vi "Unicode List Folder Example.vi"() -> ()   [LabVIEW 2020]
uses:
  Types/UTF-8 String/UTF-8 String.lvclass/UTF-8 String.ctl
  Types/UTF-8 Path/UTF-8 Path.lvclass/UTF-8 Path.ctl
  356e65d8-4da9-4114-9294-e55a313f9948.vi
  39fc5e22-d9af-4d01-836e-3ce06c2f0119.vi
  9656b7da-fab8-46cb-9ac0-8f81757845da.vi
  0798be5a-71d1-4c5d-88ab-63fcb16b67de.vi
  333a896f-bbc2-4275-b957-7d35ff018cee.vi
  d770f125-4b2e-45a9-bf4a-bdfa33aeb32b.vi
  be28db5e-b7b6-4e5e-976e-8f4788af5f3e.vi
  d890a278-da3a-47ea-bd3f-d0f581a9f8a0.vi
  e6b5bfce-c779-4612-a132-177d94a25bbe.vi
  cbe0ae27-dce3-42f5-8311-771008e4fc32.vi
  faa403f0-121f-4031-81ad-bed2ef2c299f.vi
  9acd3354-284c-4284-bd8f-25762292fedc.vi
  356e65d8-4da9-4114-9294-e55a313f9948.vi/394fe735-5a0a-4c6e-b10c-ef5f4bad8cdd.vi
  356e65d8-4da9-4114-9294-e55a313f9948.vi/c6ff4536-5c5f-4898-b0f4-ba79e0235d06.vi
  Private/Conversion/String as Encoded String.vi
  Private/Conversion/Polymorphic VIs/String as Encoded String (UTF-8 String).vi
  Types/UTF-8 String/Write Encoded UTF-8 String.vi
  39fc5e22-d9af-4d01-836e-3ce06c2f0119.vi/9afeabe8-8abe-4536-bea1-05e5a3549c28.vi
  Private/Conversion/Text as Encoded String.vi
  Private/Conversion/Polymorphic VIs/Text as Encoded String (UTF-8 String).vi
  Private/Library/gu_open_file_dialog.vi
  Private/Library/gu_select_folder_dialog.vi
  9656b7da-fab8-46cb-9ac0-8f81757845da.vi/5206cb6b-04fb-41f5-a37e-29c14f142303.vi
  0798be5a-71d1-4c5d-88ab-63fcb16b67de.vi/394fe735-5a0a-4c6e-b10c-ef5f4bad8cdd.vi
  0798be5a-71d1-4c5d-88ab-63fcb16b67de.vi/c6ff4536-5c5f-4898-b0f4-ba79e0235d06.vi
  Private/Conversion/Text as String.vi
  Private/Conversion/Polymorphic VIs/Text as String (UTF-8 String).vi
  Private/Conversion/Text as Encoded Path.vi
  Private/Conversion/Polymorphic VIs/Text as Encoded Path (UTF-8 String).vi
  Types/UTF-8 Path/Write Encoded UTF-8 Path.vi
  Private/Conversion/Path as UTF-8 Path.vi
  Private/Conversion/Polymorphic VIs/Path as UTF-8 Path (UTF-8 Path).vi
  be28db5e-b7b6-4e5e-976e-8f4788af5f3e.vi/5269e09c-4216-478e-8686-9fb7d38e224a.vi
  be28db5e-b7b6-4e5e-976e-8f4788af5f3e.vi/d1f4a45d-6f02-44dd-a40b-2b28d80e6519.vi
  Private/Library/gu_list_folder.vi
  be28db5e-b7b6-4e5e-976e-8f4788af5f3e.vi/8eb4f0ed-0012-4550-978e-be3f7301df70.vi
  be28db5e-b7b6-4e5e-976e-8f4788af5f3e.vi/f7e6584c-01ed-423f-9bcd-660954191d0d.vi
  d890a278-da3a-47ea-bd3f-d0f581a9f8a0.vi/00b95b8e-259c-4cd2-84a0-259870334f57.vi
  d890a278-da3a-47ea-bd3f-d0f581a9f8a0.vi/6e4bb66e-265d-408c-9dfe-e7c3a7878e52.vi
  d890a278-da3a-47ea-bd3f-d0f581a9f8a0.vi/08f180d4-fb41-400e-a869-abb2918b55f1.vi
  d890a278-da3a-47ea-bd3f-d0f581a9f8a0.vi/5ea8612d-ac84-4b15-a8e8-3f95405e799f.vi
  d890a278-da3a-47ea-bd3f-d0f581a9f8a0.vi/f443e8ba-b003-43b4-b0bc-fd2b779e8587.vi
  d890a278-da3a-47ea-bd3f-d0f581a9f8a0.vi/c6b89822-a9c0-4fa9-a4a0-f7d505b8bbe9.vi
  d890a278-da3a-47ea-bd3f-d0f581a9f8a0.vi/54676e99-5528-43ca-932e-9ead8464c752.vi
  d890a278-da3a-47ea-bd3f-d0f581a9f8a0.vi/9bf89ca9-aafa-4aa0-9117-a6707f6e0e94.vi
  d890a278-da3a-47ea-bd3f-d0f581a9f8a0.vi/e7542c1a-d99f-41ff-9d9a-3ecd282cacf4.vi
  d890a278-da3a-47ea-bd3f-d0f581a9f8a0.vi/d8f6ae1f-7202-4db9-b87a-1f416505b7ed.vi
  Private/Conversion/Polymorphic VIs/Text as Encoded String (UTF-8 Path).vi
  faa403f0-121f-4031-81ad-bed2ef2c299f.vi/5206cb6b-04fb-41f5-a37e-29c14f142303.vi
  9acd3354-284c-4284-bd8f-25762292fedc.vi/5206cb6b-04fb-41f5-a37e-29c14f142303.vi
  Private/Conversion/String as UTF-8 String.vi
  Private/Conversion/Polymorphic VIs/String as UTF-8 String (LabVIEW String).vi
  Types/UTF-8 String/Read Encoded UTF-8 String.vi
  Private/Memory/Copy String.vi
  Private/Library/Result To Error.vi
  be28db5e-b7b6-4e5e-976e-8f4788af5f3e.vi/5269e09c-4216-478e-8686-9fb7d38e224a.vi/c24c063b-f849-48a1-b323-238a063d7118.vi
  be28db5e-b7b6-4e5e-976e-8f4788af5f3e.vi/5269e09c-4216-478e-8686-9fb7d38e224a.vi/a2fd6c11-d594-45c9-8624-1f0a1df69df3.vi
  be28db5e-b7b6-4e5e-976e-8f4788af5f3e.vi/5269e09c-4216-478e-8686-9fb7d38e224a.vi/1fd3173e-d32e-42cb-8f0d-819132eb8e27.vi
  be28db5e-b7b6-4e5e-976e-8f4788af5f3e.vi/5269e09c-4216-478e-8686-9fb7d38e224a.vi/bb7c39fc-ad8e-447d-bc50-468674bfb562.vi
  be28db5e-b7b6-4e5e-976e-8f4788af5f3e.vi/8eb4f0ed-0012-4550-978e-be3f7301df70.vi/3a31b270-3bb6-4c58-a256-c5fcc2c98f09.vi
  be28db5e-b7b6-4e5e-976e-8f4788af5f3e.vi/8eb4f0ed-0012-4550-978e-be3f7301df70.vi/0ec5df2d-ef9b-4f84-a6a8-ffcedd45c4dc.vi
  Private/Conversion/Polymorphic VIs/Text as String (UTF-8 Path).vi
  Private/Conversion/Path as Encoded Path.vi
  Private/Conversion/Polymorphic VIs/Path as Encoded Path (UTF-8 Path).vi
  Private/Library/gu_to_lower_case.vi
  d890a278-da3a-47ea-bd3f-d0f581a9f8a0.vi/08f180d4-fb41-400e-a869-abb2918b55f1.vi/5269e09c-4216-478e-8686-9fb7d38e224a.vi
  d890a278-da3a-47ea-bd3f-d0f581a9f8a0.vi/08f180d4-fb41-400e-a869-abb2918b55f1.vi/d1f4a45d-6f02-44dd-a40b-2b28d80e6519.vi
  d890a278-da3a-47ea-bd3f-d0f581a9f8a0.vi/08f180d4-fb41-400e-a869-abb2918b55f1.vi/8eb4f0ed-0012-4550-978e-be3f7301df70.vi
  d890a278-da3a-47ea-bd3f-d0f581a9f8a0.vi/08f180d4-fb41-400e-a869-abb2918b55f1.vi/f7e6584c-01ed-423f-9bcd-660954191d0d.vi
  d890a278-da3a-47ea-bd3f-d0f581a9f8a0.vi/5ea8612d-ac84-4b15-a8e8-3f95405e799f.vi/5269e09c-4216-478e-8686-9fb7d38e224a.vi
  d890a278-da3a-47ea-bd3f-d0f581a9f8a0.vi/5ea8612d-ac84-4b15-a8e8-3f95405e799f.vi/d1f4a45d-6f02-44dd-a40b-2b28d80e6519.vi
  d890a278-da3a-47ea-bd3f-d0f581a9f8a0.vi/5ea8612d-ac84-4b15-a8e8-3f95405e799f.vi/8eb4f0ed-0012-4550-978e-be3f7301df70.vi
  d890a278-da3a-47ea-bd3f-d0f581a9f8a0.vi/5ea8612d-ac84-4b15-a8e8-3f95405e799f.vi/f7e6584c-01ed-423f-9bcd-660954191d0d.vi
  d890a278-da3a-47ea-bd3f-d0f581a9f8a0.vi/f443e8ba-b003-43b4-b0bc-fd2b779e8587.vi/bdbb2850-443b-457b-baea-a8ca465ac309.vi
  d890a278-da3a-47ea-bd3f-d0f581a9f8a0.vi/f443e8ba-b003-43b4-b0bc-fd2b779e8587.vi/12c50203-b387-4b7f-a219-1cc37bee024e.vi
  d890a278-da3a-47ea-bd3f-d0f581a9f8a0.vi/f443e8ba-b003-43b4-b0bc-fd2b779e8587.vi/79db7a21-11bb-4b22-98c5-d1966ec86c45.vi
  d890a278-da3a-47ea-bd3f-d0f581a9f8a0.vi/f443e8ba-b003-43b4-b0bc-fd2b779e8587.vi/90888b97-91dc-4a8b-9ef5-bc117a67dfd4.vi
  d890a278-da3a-47ea-bd3f-d0f581a9f8a0.vi/f443e8ba-b003-43b4-b0bc-fd2b779e8587.vi/1e320fb2-7d21-4fd0-8d77-02d925575486.vi
  d890a278-da3a-47ea-bd3f-d0f581a9f8a0.vi/f443e8ba-b003-43b4-b0bc-fd2b779e8587.vi/3a50a1cc-fee8-47d0-b63a-e1c29b38961d.vi
  d890a278-da3a-47ea-bd3f-d0f581a9f8a0.vi/54676e99-5528-43ca-932e-9ead8464c752.vi/4d3f9d4a-5006-44fd-9ac3-fe6a2ce0b86b.vi
  d890a278-da3a-47ea-bd3f-d0f581a9f8a0.vi/54676e99-5528-43ca-932e-9ead8464c752.vi/29e5914f-c0b0-4539-b998-9919647c2bfd.vi
  d890a278-da3a-47ea-bd3f-d0f581a9f8a0.vi/9bf89ca9-aafa-4aa0-9117-a6707f6e0e94.vi/4d3f9d4a-5006-44fd-9ac3-fe6a2ce0b86b.vi
  d890a278-da3a-47ea-bd3f-d0f581a9f8a0.vi/9bf89ca9-aafa-4aa0-9117-a6707f6e0e94.vi/29e5914f-c0b0-4539-b998-9919647c2bfd.vi
  Types/UTF-8 Path/Read Encoded UTF-8 Path.vi
  Types/UTF-8 String/New UTF-8 String.vi
  Private/Memory/Copy String.vi/4d47babd-4a2d-4eb7-b91b-7e707d692665.vi
  Private/Library/gu_free.vi
  Private/Library/gu_string_subset.vi
  Private/Library/gu_search_split_string.vi
  Private/Conversion/Polymorphic VIs/String as Encoded String (LabVIEW String).vi
  Private/Conversion/Polymorphic VIs/Text as Encoded String (LabVIEW String).vi
  d890a278-da3a-47ea-bd3f-d0f581a9f8a0.vi/08f180d4-fb41-400e-a869-abb2918b55f1.vi/5269e09c-4216-478e-8686-9fb7d38e224a.vi/c24c063b-f849-48a1-b323-238a063d7118.vi
  d890a278-da3a-47ea-bd3f-d0f581a9f8a0.vi/08f180d4-fb41-400e-a869-abb2918b55f1.vi/5269e09c-4216-478e-8686-9fb7d38e224a.vi/a2fd6c11-d594-45c9-8624-1f0a1df69df3.vi
  d890a278-da3a-47ea-bd3f-d0f581a9f8a0.vi/08f180d4-fb41-400e-a869-abb2918b55f1.vi/5269e09c-4216-478e-8686-9fb7d38e224a.vi/1fd3173e-d32e-42cb-8f0d-819132eb8e27.vi
  d890a278-da3a-47ea-bd3f-d0f581a9f8a0.vi/08f180d4-fb41-400e-a869-abb2918b55f1.vi/5269e09c-4216-478e-8686-9fb7d38e224a.vi/bb7c39fc-ad8e-447d-bc50-468674bfb562.vi
  d890a278-da3a-47ea-bd3f-d0f581a9f8a0.vi/08f180d4-fb41-400e-a869-abb2918b55f1.vi/8eb4f0ed-0012-4550-978e-be3f7301df70.vi/3a31b270-3bb6-4c58-a256-c5fcc2c98f09.vi
  d890a278-da3a-47ea-bd3f-d0f581a9f8a0.vi/08f180d4-fb41-400e-a869-abb2918b55f1.vi/8eb4f0ed-0012-4550-978e-be3f7301df70.vi/0ec5df2d-ef9b-4f84-a6a8-ffcedd45c4dc.vi
  d890a278-da3a-47ea-bd3f-d0f581a9f8a0.vi/5ea8612d-ac84-4b15-a8e8-3f95405e799f.vi/5269e09c-4216-478e-8686-9fb7d38e224a.vi/c24c063b-f849-48a1-b323-238a063d7118.vi
  d890a278-da3a-47ea-bd3f-d0f581a9f8a0.vi/5ea8612d-ac84-4b15-a8e8-3f95405e799f.vi/5269e09c-4216-478e-8686-9fb7d38e224a.vi/a2fd6c11-d594-45c9-8624-1f0a1df69df3.vi
  d890a278-da3a-47ea-bd3f-d0f581a9f8a0.vi/5ea8612d-ac84-4b15-a8e8-3f95405e799f.vi/5269e09c-4216-478e-8686-9fb7d38e224a.vi/1fd3173e-d32e-42cb-8f0d-819132eb8e27.vi
  d890a278-da3a-47ea-bd3f-d0f581a9f8a0.vi/5ea8612d-ac84-4b15-a8e8-3f95405e799f.vi/5269e09c-4216-478e-8686-9fb7d38e224a.vi/bb7c39fc-ad8e-447d-bc50-468674bfb562.vi
  d890a278-da3a-47ea-bd3f-d0f581a9f8a0.vi/5ea8612d-ac84-4b15-a8e8-3f95405e799f.vi/8eb4f0ed-0012-4550-978e-be3f7301df70.vi/3a31b270-3bb6-4c58-a256-c5fcc2c98f09.vi
  d890a278-da3a-47ea-bd3f-d0f581a9f8a0.vi/5ea8612d-ac84-4b15-a8e8-3f95405e799f.vi/8eb4f0ed-0012-4550-978e-be3f7301df70.vi/0ec5df2d-ef9b-4f84-a6a8-ffcedd45c4dc.vi
  d890a278-da3a-47ea-bd3f-d0f581a9f8a0.vi/f443e8ba-b003-43b4-b0bc-fd2b779e8587.vi/90888b97-91dc-4a8b-9ef5-bc117a67dfd4.vi/5269e09c-4216-478e-8686-9fb7d38e224a.vi
  d890a278-da3a-47ea-bd3f-d0f581a9f8a0.vi/f443e8ba-b003-43b4-b0bc-fd2b779e8587.vi/90888b97-91dc-4a8b-9ef5-bc117a67dfd4.vi/d1f4a45d-6f02-44dd-a40b-2b28d80e6519.vi
  d890a278-da3a-47ea-bd3f-d0f581a9f8a0.vi/f443e8ba-b003-43b4-b0bc-fd2b779e8587.vi/90888b97-91dc-4a8b-9ef5-bc117a67dfd4.vi/8eb4f0ed-0012-4550-978e-be3f7301df70.vi
  d890a278-da3a-47ea-bd3f-d0f581a9f8a0.vi/f443e8ba-b003-43b4-b0bc-fd2b779e8587.vi/90888b97-91dc-4a8b-9ef5-bc117a67dfd4.vi/f7e6584c-01ed-423f-9bcd-660954191d0d.vi
  d890a278-da3a-47ea-bd3f-d0f581a9f8a0.vi/f443e8ba-b003-43b4-b0bc-fd2b779e8587.vi/1e320fb2-7d21-4fd0-8d77-02d925575486.vi/5269e09c-4216-478e-8686-9fb7d38e224a.vi
  d890a278-da3a-47ea-bd3f-d0f581a9f8a0.vi/f443e8ba-b003-43b4-b0bc-fd2b779e8587.vi/1e320fb2-7d21-4fd0-8d77-02d925575486.vi/d1f4a45d-6f02-44dd-a40b-2b28d80e6519.vi
  d890a278-da3a-47ea-bd3f-d0f581a9f8a0.vi/f443e8ba-b003-43b4-b0bc-fd2b779e8587.vi/1e320fb2-7d21-4fd0-8d77-02d925575486.vi/8eb4f0ed-0012-4550-978e-be3f7301df70.vi
  d890a278-da3a-47ea-bd3f-d0f581a9f8a0.vi/f443e8ba-b003-43b4-b0bc-fd2b779e8587.vi/1e320fb2-7d21-4fd0-8d77-02d925575486.vi/f7e6584c-01ed-423f-9bcd-660954191d0d.vi
  d890a278-da3a-47ea-bd3f-d0f581a9f8a0.vi/f443e8ba-b003-43b4-b0bc-fd2b779e8587.vi/3a50a1cc-fee8-47d0-b63a-e1c29b38961d.vi/5269e09c-4216-478e-8686-9fb7d38e224a.vi
  d890a278-da3a-47ea-bd3f-d0f581a9f8a0.vi/f443e8ba-b003-43b4-b0bc-fd2b779e8587.vi/3a50a1cc-fee8-47d0-b63a-e1c29b38961d.vi/d1f4a45d-6f02-44dd-a40b-2b28d80e6519.vi
  d890a278-da3a-47ea-bd3f-d0f581a9f8a0.vi/f443e8ba-b003-43b4-b0bc-fd2b779e8587.vi/3a50a1cc-fee8-47d0-b63a-e1c29b38961d.vi/8eb4f0ed-0012-4550-978e-be3f7301df70.vi
  d890a278-da3a-47ea-bd3f-d0f581a9f8a0.vi/f443e8ba-b003-43b4-b0bc-fd2b779e8587.vi/3a50a1cc-fee8-47d0-b63a-e1c29b38961d.vi/f7e6584c-01ed-423f-9bcd-660954191d0d.vi
  Private/Conversion/Text to UTF-8.vi
  Private/Conversion/Polymorphic VIs/Text to UTF-8 (LabVIEW String).vi
  d890a278-da3a-47ea-bd3f-d0f581a9f8a0.vi/f443e8ba-b003-43b4-b0bc-fd2b779e8587.vi/90888b97-91dc-4a8b-9ef5-bc117a67dfd4.vi/5269e09c-4216-478e-8686-9fb7d38e224a.vi/c24c063b-f849-48a1-b323-238a063d7118.vi
  d890a278-da3a-47ea-bd3f-d0f581a9f8a0.vi/f443e8ba-b003-43b4-b0bc-fd2b779e8587.vi/90888b97-91dc-4a8b-9ef5-bc117a67dfd4.vi/5269e09c-4216-478e-8686-9fb7d38e224a.vi/a2fd6c11-d594-45c9-8624-1f0a1df69df3.vi
  d890a278-da3a-47ea-bd3f-d0f581a9f8a0.vi/f443e8ba-b003-43b4-b0bc-fd2b779e8587.vi/90888b97-91dc-4a8b-9ef5-bc117a67dfd4.vi/5269e09c-4216-478e-8686-9fb7d38e224a.vi/1fd3173e-d32e-42cb-8f0d-819132eb8e27.vi
  d890a278-da3a-47ea-bd3f-d0f581a9f8a0.vi/f443e8ba-b003-43b4-b0bc-fd2b779e8587.vi/90888b97-91dc-4a8b-9ef5-bc117a67dfd4.vi/5269e09c-4216-478e-8686-9fb7d38e224a.vi/bb7c39fc-ad8e-447d-bc50-468674bfb562.vi
  d890a278-da3a-47ea-bd3f-d0f581a9f8a0.vi/f443e8ba-b003-43b4-b0bc-fd2b779e8587.vi/90888b97-91dc-4a8b-9ef5-bc117a67dfd4.vi/8eb4f0ed-0012-4550-978e-be3f7301df70.vi/3a31b270-3bb6-4c58-a256-c5fcc2c98f09.vi
  d890a278-da3a-47ea-bd3f-d0f581a9f8a0.vi/f443e8ba-b003-43b4-b0bc-fd2b779e8587.vi/90888b97-91dc-4a8b-9ef5-bc117a67dfd4.vi/8eb4f0ed-0012-4550-978e-be3f7301df70.vi/0ec5df2d-ef9b-4f84-a6a8-ffcedd45c4dc.vi
  d890a278-da3a-47ea-bd3f-d0f581a9f8a0.vi/f443e8ba-b003-43b4-b0bc-fd2b779e8587.vi/1e320fb2-7d21-4fd0-8d77-02d925575486.vi/5269e09c-4216-478e-8686-9fb7d38e224a.vi/c24c063b-f849-48a1-b323-238a063d7118.vi
  d890a278-da3a-47ea-bd3f-d0f581a9f8a0.vi/f443e8ba-b003-43b4-b0bc-fd2b779e8587.vi/1e320fb2-7d21-4fd0-8d77-02d925575486.vi/5269e09c-4216-478e-8686-9fb7d38e224a.vi/a2fd6c11-d594-45c9-8624-1f0a1df69df3.vi
  d890a278-da3a-47ea-bd3f-d0f581a9f8a0.vi/f443e8ba-b003-43b4-b0bc-fd2b779e8587.vi/1e320fb2-7d21-4fd0-8d77-02d925575486.vi/5269e09c-4216-478e-8686-9fb7d38e224a.vi/1fd3173e-d32e-42cb-8f0d-819132eb8e27.vi
  d890a278-da3a-47ea-bd3f-d0f581a9f8a0.vi/f443e8ba-b003-43b4-b0bc-fd2b779e8587.vi/1e320fb2-7d21-4fd0-8d77-02d925575486.vi/5269e09c-4216-478e-8686-9fb7d38e224a.vi/bb7c39fc-ad8e-447d-bc50-468674bfb562.vi
  d890a278-da3a-47ea-bd3f-d0f581a9f8a0.vi/f443e8ba-b003-43b4-b0bc-fd2b779e8587.vi/1e320fb2-7d21-4fd0-8d77-02d925575486.vi/8eb4f0ed-0012-4550-978e-be3f7301df70.vi/3a31b270-3bb6-4c58-a256-c5fcc2c98f09.vi
  d890a278-da3a-47ea-bd3f-d0f581a9f8a0.vi/f443e8ba-b003-43b4-b0bc-fd2b779e8587.vi/1e320fb2-7d21-4fd0-8d77-02d925575486.vi/8eb4f0ed-0012-4550-978e-be3f7301df70.vi/0ec5df2d-ef9b-4f84-a6a8-ffcedd45c4dc.vi
  d890a278-da3a-47ea-bd3f-d0f581a9f8a0.vi/f443e8ba-b003-43b4-b0bc-fd2b779e8587.vi/3a50a1cc-fee8-47d0-b63a-e1c29b38961d.vi/5269e09c-4216-478e-8686-9fb7d38e224a.vi/c24c063b-f849-48a1-b323-238a063d7118.vi
  d890a278-da3a-47ea-bd3f-d0f581a9f8a0.vi/f443e8ba-b003-43b4-b0bc-fd2b779e8587.vi/3a50a1cc-fee8-47d0-b63a-e1c29b38961d.vi/5269e09c-4216-478e-8686-9fb7d38e224a.vi/a2fd6c11-d594-45c9-8624-1f0a1df69df3.vi
  d890a278-da3a-47ea-bd3f-d0f581a9f8a0.vi/f443e8ba-b003-43b4-b0bc-fd2b779e8587.vi/3a50a1cc-fee8-47d0-b63a-e1c29b38961d.vi/5269e09c-4216-478e-8686-9fb7d38e224a.vi/1fd3173e-d32e-42cb-8f0d-819132eb8e27.vi
  d890a278-da3a-47ea-bd3f-d0f581a9f8a0.vi/f443e8ba-b003-43b4-b0bc-fd2b779e8587.vi/3a50a1cc-fee8-47d0-b63a-e1c29b38961d.vi/5269e09c-4216-478e-8686-9fb7d38e224a.vi/bb7c39fc-ad8e-447d-bc50-468674bfb562.vi
  d890a278-da3a-47ea-bd3f-d0f581a9f8a0.vi/f443e8ba-b003-43b4-b0bc-fd2b779e8587.vi/3a50a1cc-fee8-47d0-b63a-e1c29b38961d.vi/8eb4f0ed-0012-4550-978e-be3f7301df70.vi/3a31b270-3bb6-4c58-a256-c5fcc2c98f09.vi
  d890a278-da3a-47ea-bd3f-d0f581a9f8a0.vi/f443e8ba-b003-43b4-b0bc-fd2b779e8587.vi/3a50a1cc-fee8-47d0-b63a-e1c29b38961d.vi/8eb4f0ed-0012-4550-978e-be3f7301df70.vi/0ec5df2d-ef9b-4f84-a6a8-ffcedd45c4dc.vi
  Private/User Interface/Read String.vi
  Unicode/Detect String Encoding.vi
  Private/Conversion/Encoded UTF-16LE String to Encoded UTF-8 String.vi
  <vilib>/Utility/error.llb/Error Cluster From Error Code.vi
  Private/Conversion/Encoded UTF-8 String to Encoded UTF-16LE String.vi
  Private/User Interface/Write String.vi
  Private/Memory/Copy String Array.vi
  File IO/Path to Short Name.vi
  Private/Library/gu_strlen.vi
  Private/User Interface/Write String Array (1D).vi
  Types/UTF-8 String/UTF-8 String.lvclass
  Types/UTF-8 Path/UTF-8 Path.lvclass
panel:
  in  "Refresh Button":bool
  in  "Recursive List":bool
  out "Files":string[](array[string])
  out "Folders":string[](array[string])
  in  "Browse Button":bool
  out "Path":string
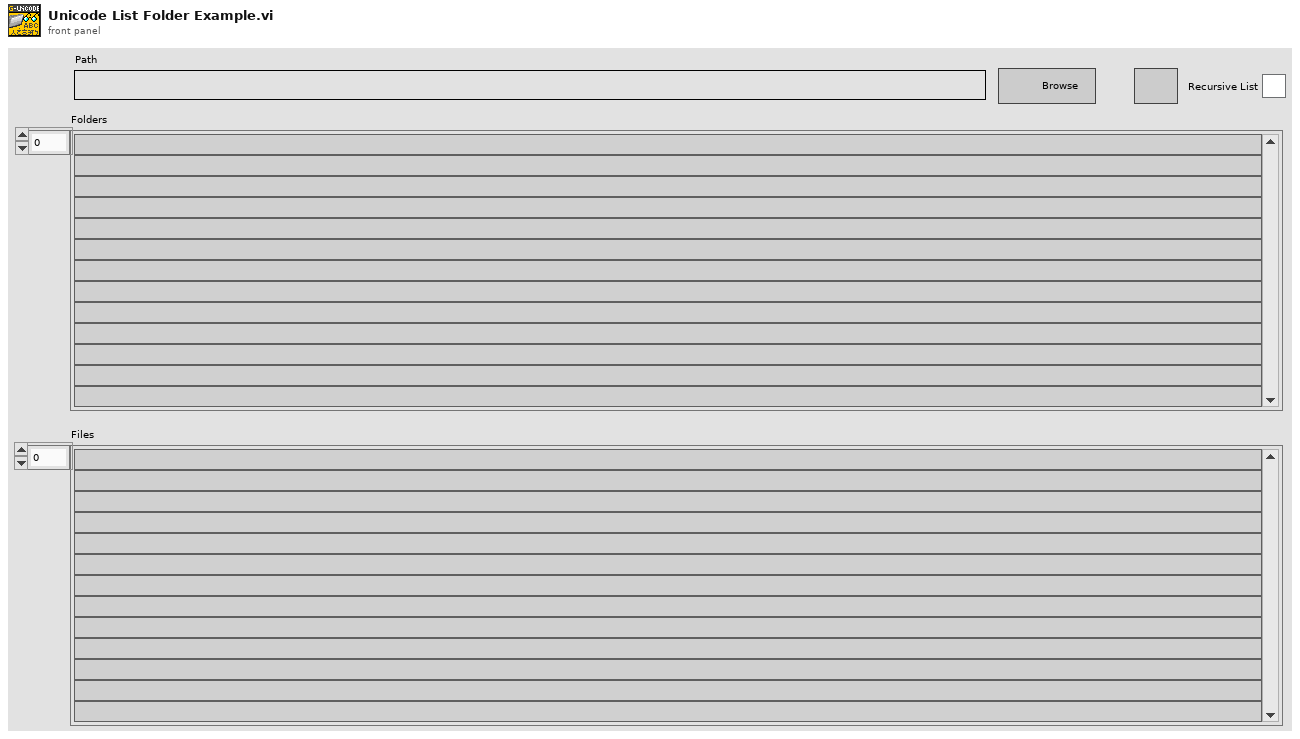
[diagram p1: front panel]
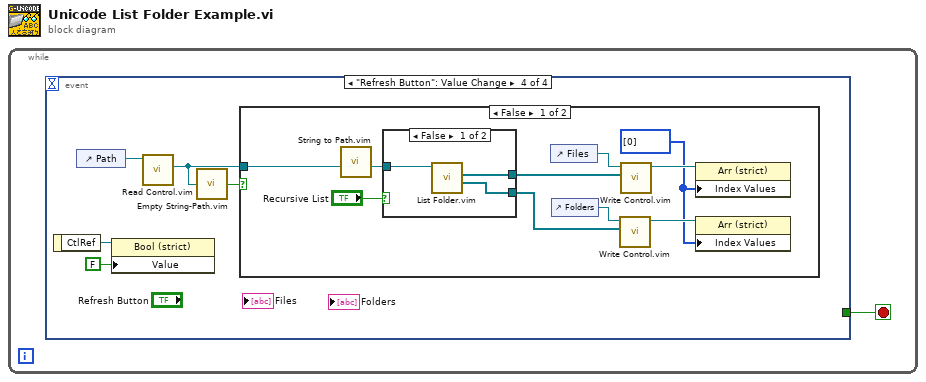
[diagram p0: block diagram]
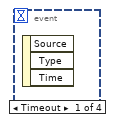
[diagram p2: hidden frame]
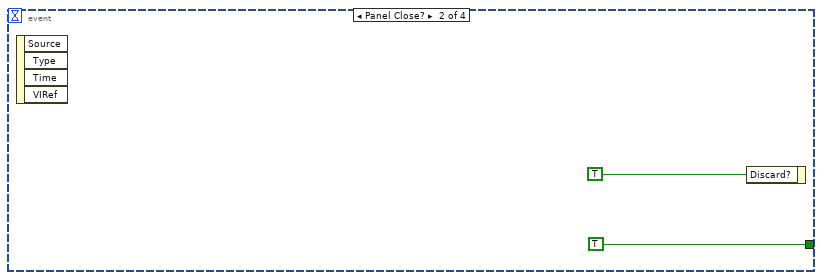
[diagram p3: hidden frame]
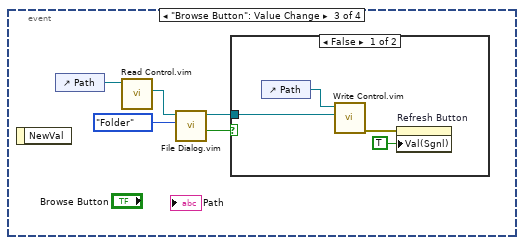
[diagram p4: hidden frame]
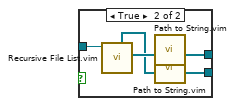
[diagram p6: hidden frame]
diagram:
  n1 = while {
    stop <- w1 stop-if-true
    n2 = event shown="[3] \"Refresh Button\": Value Change" {
      selector: _ -> [_ _ _ _]
      dyn-events: _ -> [_ _ _ _]
      timeout: _ -> [_ _ _ _]
      tunnel: [_ TRUE _ _] -> w1
      event Timeout {
        n3 = event-data() -> ()  [unwired: 1 in, 3 out]
      }
      event Panel Close? {
        n4 = event-data() -> ()  [unwired: 1 in, 4 out]
        n5 = event-data("Discard?"=TRUE) -> ()  [unwired: 1 in, 1 out]
      }
      event "Browse Button": Value Change {
        n6 = event-data() -> ()  [unwired: 1 in, 1 out]
        n7 = control-ref of="Path"() -> (w5:refnum<vi>)
        n8 = call "Read Control.vim"("Control Ref"=w5) -> ("UTF-8 String"=w4:refnum<class "UTF-8 String.lvclass">)  [unwired: 8 in, 2 out]
        n9 = call "File Dialog.vim"("Selection"=enum16{"File", "Multiple Files", "Folder"}."Folder", "Start Path"=w4) -> ("Cancelled"=w7:bool, "Selected Path"=w8:refnum<class "UTF-8 Path.lvclass">)  [unwired: 7 in, 1 out]
        n10 = case shown="False" w7 {
          tunnel: w8 -> [w9 _]
          frame False {
            n11 = control-ref of="Path"() -> (w12:refnum<vi>)
            n12 = call "Write Control.vim"("Text"=w9, "Control Ref"=w12) -> ("error out"=w11:errorcluster)  [unwired: 8 in, 1 out]
            n13 = property on="Refresh Button" class="Bool (strict)"(error in=w11, "Val(Sgnl)"=TRUE ("Value (Signaling)")) -> ()  [unwired: 1 in, 2 out]
          }
          frame True {
          }
        }
      }
      event "Refresh Button": Value Change {
        n14 = event-data() -> ("CtlRef"=w17:refnum<vi>)  [unwired: 1 in]
        n15 = control-ref of="Path"() -> (w13:refnum<vi>)
        n16 = property class="Bool (strict)"(reference=w17, "Value"=FALSE) -> ()  [unwired: 1 in, 2 out]
        n17 = call "Read Control.vim"("Control Ref"=w13) -> ("UTF-8 String"=w15:refnum<class "UTF-8 String.lvclass">)  [unwired: 8 in, 2 out]
        n18 = call "Empty String-Path.vim"("String/Path"=w15) -> ("Empty?"=w14:bool)
        n19 = case shown="False" w14 {
          tunnel: w15 -> [w21 _]
          frame False {
            w18 = u32[] [0] ("Index Values")
            n20 = call "String to Path.vim"("String"=w21) -> ("Path"=w22:refnum<class "UTF-8 Path.lvclass">)  [unwired: 9 in, 1 out]
            n21 = case shown="False" "Recursive List" {
              tunnel: [w30 w34] -> w26
              tunnel: [w29 w32] -> w24
              tunnel: w22 -> [w28 w31]
              frame False {
                n22 = call "List Folder.vim"("Path"=w28) -> ("Folder Names"=w29:refnum<class "UTF-8 String.lvclass">[], "Filenames"=w30:refnum<class "UTF-8 String.lvclass">[])  [unwired: 7 in, 2 out]
              }
              frame True {
                n23 = call "Recursive File List.vim"("Folder Path"=w31) -> ("All Files in Dir"=w35:refnum<class "UTF-8 Path.lvclass">[], "All Folders"=w33:refnum<class "UTF-8 Path.lvclass">[])  [unwired: 6 in, 3 out]
                n24 = call "Path to String.vim"("Path"=w35) -> ("String"=w34:refnum<class "UTF-8 String.lvclass">[])  [unwired: 9 in, 1 out]
                n25 = call "Path to String.vim"("Path"=w33) -> ("String"=w32:refnum<class "UTF-8 String.lvclass">[])  [unwired: 9 in, 1 out]
              }
            }
            n26 = control-ref of="Files"() -> (w25:refnum<vi>)
            n27 = control-ref of="Folders"() -> (w23:refnum<vi>)
            n28 = call "Write Control.vim"("Text"=w24, "Control Ref"=w23) -> ("Control Ref dup"=w19:refnum<vi>)  [unwired: 8 in, 1 out]
            n29 = call "Write Control.vim"("Text"=w26, "Control Ref"=w25) -> ("Control Ref dup"=w20:refnum<vi>)  [unwired: 8 in, 1 out]
            n30 = property class="Arr (strict)"(reference=w20, "Index Values"=w18) -> ()  [unwired: 1 in, 2 out]
            n31 = property class="Arr (strict)"(reference=w19, "Index Values"=w18) -> ()  [unwired: 1 in, 2 out]
          }
          frame True {
          }
        }
      }
    }
  }
